vi "FPGAPowerMeasurementSaveData.vi"(2 "rate":dbl=2000000.0, 3 "number of samples":i32=2000000, 4 "timeout (s)":dbl=10.0 format="%0.2f", 5 "error in":errorcluster, 7 "stop (T)":bool=TRUE) -> (14 "task out":refnum<k21>, 15 "data":dynamicdata(graph), 19 "error out":errorcluster)   [LabVIEW 2009]
doc: "Creates, edits, and runs tasks using NI-DAQmx. Refer to the NI-DAQmx Readme for a complete listing of devices NI-DAQmx supports.\n\nWhen you place this Express VI on the block diagram, the DAQ Assistant launches to create a new task. After you create a task, you can double-click the DAQ Assistant Express VI to edit that task. For continuous measurement or generation, place a while loop around the DAQ Assistant Express VI.\n\nFor continuous single-point input or output, the DAQ Assistant Express VI might not provide optimal performance. Refer to the Cont Acq&Graph Voltage-Single Point Optimization VI in examples\\DAQmx\\Analog In\\Measure Voltage.llb for an example of techniques to create higher-performance, single-point I/O applications."
uses:
  <vilib>/DAQmx/read.llb/DAQmx Read.vi
  <vilib>/DAQmx/read.llb/DAQmx Read (Analog 1D Wfm NChan NSamp).vi
  <vilib>/DAQmx/create/channels.llb/DAQmx Create Channel (TEDS-AI-Voltage-Basic).vi
  <vilib>/DAQmx/create/channels.llb/DAQmx Create Channel (AI-Voltage-Basic).vi
  <vilib>/DAQmx/configure/timing.llb/DAQmx Timing (Sample Clock).vi
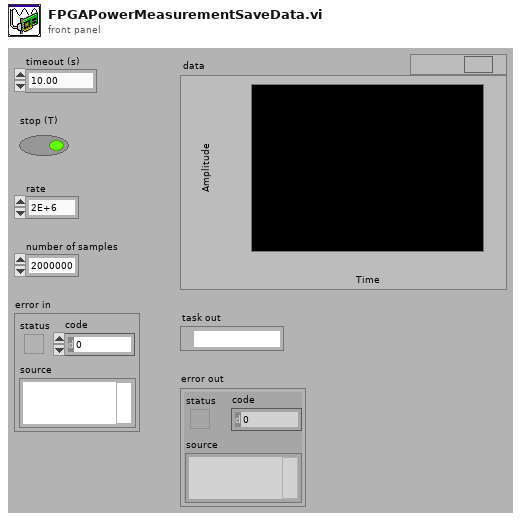
[diagram p1: front panel]
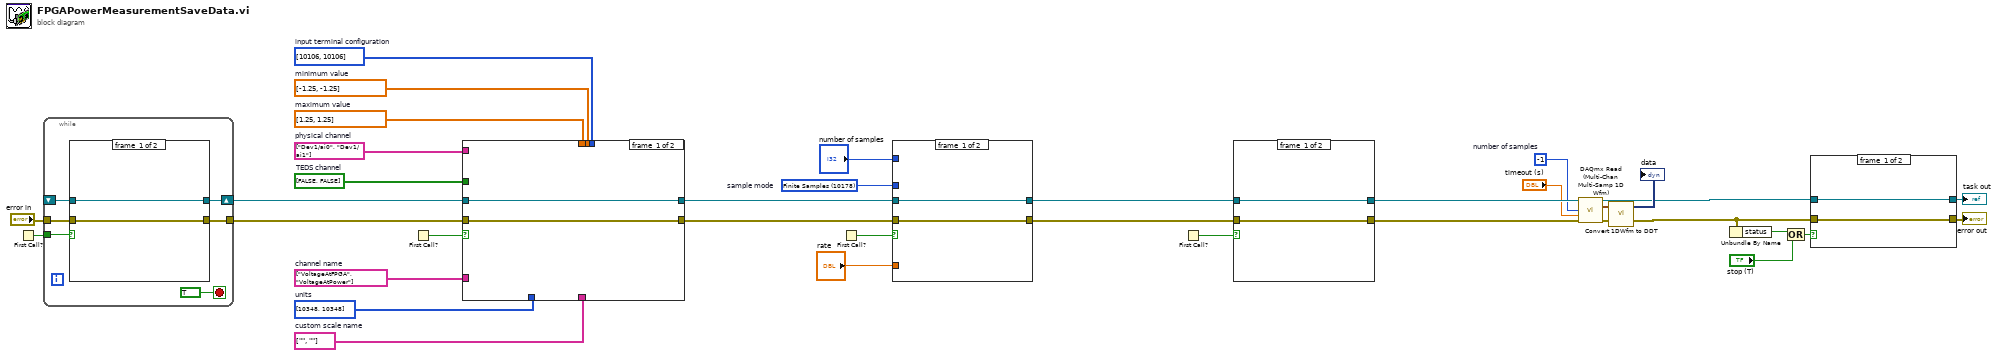
[diagram p0: block diagram]
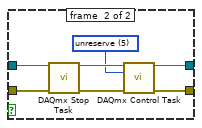
[diagram p2: hidden frame]
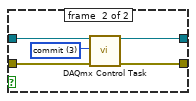
[diagram p3: hidden frame]
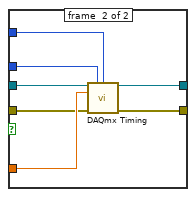
[diagram p4: hidden frame]
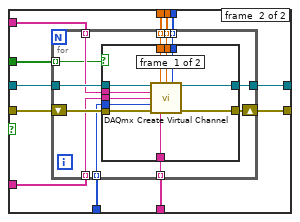
[diagram p5: hidden frame]
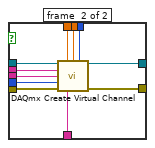
[diagram p6: hidden frame]
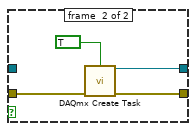
[diagram p7: hidden frame]
diagram:
  w10 = -1  # number of samples
  w16 = 10178 items=["Finite Samples"=10178, "Continuous Samples"=10123, "Hardware Timed Single Point"=12522]  # sample mode
  w22 = bool[] [FALSE, FALSE]  # TEDS channel
  w23 = string[] ["", ""]  # custom scale name
  w24 = i32[] [10348, 10348] items=["Volts"=10348, "From TEDS"=12516, "From Custom Scale"=10065]  # units
  w25 = string[] ["VoltageAtFPGA", "VoltageAtPower"]  # channel name
  w26 = string[] ["Dev1/ai0", "Dev1/ai1"]  # physical channel
  w27 = dbl[] [1.25, 1.25]  # maximum value
  w28 = dbl[] [-1.25, -1.25]  # minimum value
  w29 = i32[] [10106, 10106] items=["default"=-1, "RSE"=10083, "NRSE"=10078, "Differential"=10106, "Pseudodifferential"=12529]  # input terminal configuration
  n1 = First Call?() -> (First Call?: T/F=w35:bool)
  n2 = while {
    shift-right: [w40] -> w31
    shift-left: _ -> [w39]
    tunnel: w35 -> [w41]
    tunnel: [w38] -> w34
    tunnel: "error in" -> [w37]
    stop <- TRUE stop-if-true
    n3 = case shown="True" w41 {
      tunnel: [w43 w47] -> w40
      tunnel: w39 -> [w43 _]
      tunnel: [w42 w46] -> w38
      tunnel: w37 -> [w42 w44]
      frame #0 {
      }
      frame #1 {
        n4 = call <vilib>:"DAQmx Create Task.vi"("auto cleanup"=TRUE, "error in"=w44) -> ("task out"=w47:refnum<k21>, "error out"=w46:errorcluster)  [unwired: 12 in]
      }
    }
  }
  n5 = First Call?() -> (First Call?: T/F=w32:bool)
  n6 = case shown="True" w32 {
    tunnel: [w49 w59] -> w20
    tunnel: w31 -> [w49 w61]
    tunnel: [w48 w58] -> w30
    tunnel: w34 -> [w48 w60]
    tunnel: w29 -> [_ w57]
    tunnel: w28 -> [_ w56]
    tunnel: w27 -> [_ w55]
    tunnel: w26 -> [_ w54]
    tunnel: w25 -> [_ w53]
    tunnel: w24 -> [_ w52]
    tunnel: w23 -> [_ w51]
    tunnel: w22 -> [_ w50]
    frame #0 {
    }
    frame #1 {
      n7 = for {
        tunnel: w61 -> [w73]
        tunnel: [w71] -> w59
        tunnel: w57 -> [w69] mode=indexing
        tunnel: w56 -> [w68] mode=indexing
        tunnel: w55 -> [w67] mode=indexing
        tunnel: w54 -> [w66] mode=indexing
        tunnel: w53 -> [w65] mode=indexing
        tunnel: w52 -> [w64] mode=indexing
        tunnel: w51 -> [w63] mode=indexing
        shift-right: [w70] -> w58
        shift-left: w60 -> [w72]
        tunnel: w50 -> [w62] mode=indexing
        n8 = case shown="False" w62 {
          tunnel: w73 -> [w84 w95]
          tunnel: w72 -> [w83 w94]
          tunnel: [w82 w93] -> w71
          tunnel: [w81 w92] -> w70
          tunnel: w69 -> [w80 w91]
          tunnel: w68 -> [w79 w90]
          tunnel: w67 -> [w78 w89]
          tunnel: w66 -> [w77 w88]
          tunnel: w65 -> [w76 w87]
          tunnel: w64 -> [w75 w86]
          tunnel: w63 -> [w74 w85]
          frame #0 {
            n9 = call-poly <vilib>:"DAQmx Create Virtual Channel.vi"("task in"=w84, "maximum value"=w78, "minimum value"=w79, "input terminal configuration"=w80, "physical channels"=w77, "name to assign"=w76, "units"=w75, "error in"=w83, "custom scale name"=w74) -> ("task out"=w82:refnum<k21>, "error out"=w81:errorcluster)  [unwired: 5 in]
          }
          frame #1 {
            n10 = call-poly <vilib>:"DAQmx Create Virtual Channel.vi"("task in"=w95, "maximum value"=w89, "minimum value"=w90, "input terminal configuration"=w91, "physical channels"=w88, "name to assign"=w87, "units"=w86, "error in"=w94, "custom scale name"=w85) -> ("task out"=w93:refnum<k21>, "error out"=w92:errorcluster)  [unwired: 5 in]
          }
        }
      }
    }
  }
  n11 = First Call?() -> (First Call?: T/F=w21:bool)
  n12 = case shown="True" w21 {
    tunnel: [w97 w99] -> w14
    tunnel: w20 -> [w97 w102]
    tunnel: [w96 w98] -> w19
    tunnel: w30 -> [w96 w100]
    tunnel: "number of samples" -> [_ w104]
    tunnel: w16 -> [_ w103]
    tunnel: "rate" -> [_ w101]
    frame #0 {
    }
    frame #1 {
      n13 = call-poly <vilib>:"DAQmx Timing.vi"("task/channels in"=w102, "sample mode"=w103, "samples per channel"=w104, "rate"=w101, "error in"=w100) -> ("task out"=w99:refnum<k21>, "error out"=w98:errorcluster)  [unwired: 9 in]
    }
  }
  n14 = First Call?() -> (First Call?: T/F=w15:bool)
  n15 = case shown="True" w15 {
    tunnel: [w106 w110] -> w11
    tunnel: w14 -> [w106 w111]
    tunnel: [w105 w108] -> w13
    tunnel: w19 -> [w105 w109]
    frame #0 {
    }
    frame #1 {
      w107 = 3 items=["verify"=2, "reserve"=4, "commit"=3, "unreserve"=5, "abort"=6] ("action")
      n16 = call <vilib>:"DAQmx Control Task.vi"("task/channels in"=w111, "action"=w107, "error in"=w109) -> ("task out"=w110:refnum<k21>, "error out"=w108:errorcluster)  [unwired: 11 in]
    }
  }
  n17 = call-poly "DAQmx Read (Multi-Chan Multi-Samp 1D Wfm).vi"("task/channels in"=w11, "number of samples per channel"=w10, "timeout"="timeout (s)", "error in"=w13) -> ("task out"=w5:refnum<k21>, "data"=w9:waveform(dbl)[], "error out"=w12:errorcluster)  [unwired: 9 in]
  n18 = call <vilib>:"Convert 1DWfm to DDT.vi"("Array of Waveforms"=w9) -> ("Dynamic Data Type"=→"data":dynamicdata)  [unwired: 3 in]
  n19 = Unbundle By Name(w12) -> ("status"=w3:bool)
  n20 = Or(x=w3, y="stop (T)") -> (x .or. y?=w1:bool)
  n21 = case shown="True" w1 {
    tunnel: [w113 w114] -> w6
    tunnel: w5 -> [w113 w120]
    tunnel: [w112 w117] -> w4
    tunnel: w12 -> [w112 w119]
    frame #0 {
    }
    frame #1 {
      w115 = 5 items=["verify"=2, "reserve"=4, "commit"=3, "unreserve"=5, "abort"=6] ("action")
      n22 = call <vilib>:"DAQmx Stop Task.vi"("task/channels in"=w120, "error in"=w119) -> ("task out"=w116:refnum<k21>, "error out"=w118:errorcluster)  [unwired: 12 in]
      n23 = call <vilib>:"DAQmx Control Task.vi"("task/channels in"=w116, "action"=w115, "error in"=w118) -> ("task out"=w114:refnum<k21>, "error out"=w117:errorcluster)  [unwired: 11 in]
    }
  }
  "task out" <- w6
  "error out" <- w4
